vi "Shutdown HW.vi"(8 "error in (no error)":errorcluster, 11 "Simulated Force Sensor in":refnum<class "Simulated Force Sensor.lvclass">) -> (0 "error out":errorcluster, 3 "Simulated Force Sensor out":refnum<class "Simulated Force Sensor.lvclass">)   [LabVIEW 2020, in "Simulated Force Sensor.lvclass"]
uses:
  Simulated Force Sensor.lvclass
  Force Sensor.lvclass
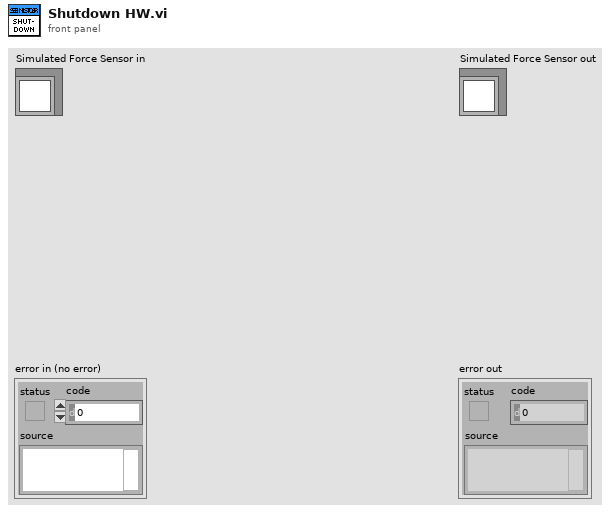
[diagram p1: front panel]
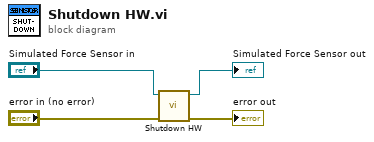
[diagram p0: block diagram]
diagram:
  n1 = call-parent "Shutdown HW.vi"("error in (no error)"="error in (no error)", "Force Sensor in"="Simulated Force Sensor in") -> ("error out"=→"error out":errorcluster, "Force Sensor out"=→"Simulated Force Sensor out":refnum<class "Simulated Force Sensor.lvclass">)  [unwired: 8 in]
